vi "ADCP_write_packet_to_serial_port.vi"(8 "error in (no error)":errorcluster, 10 "Packet Bytes":u8[](array[numeric]), 11 "ADCP In":refnum<class "ADCP.lvclass">) -> (0 "error out":errorcluster, 3 "ADCP Out":refnum<class "ADCP.lvclass">)   [LabVIEW 2017, in "ADCP.lvclass"]
uses:
  ADCP.lvclass
  ADCP.lvclass/ADCP.ctl
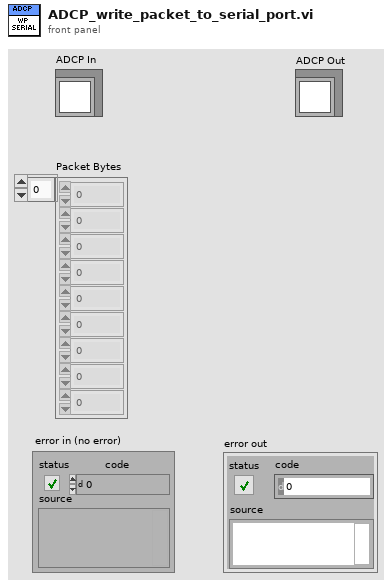
[diagram p1: front panel]
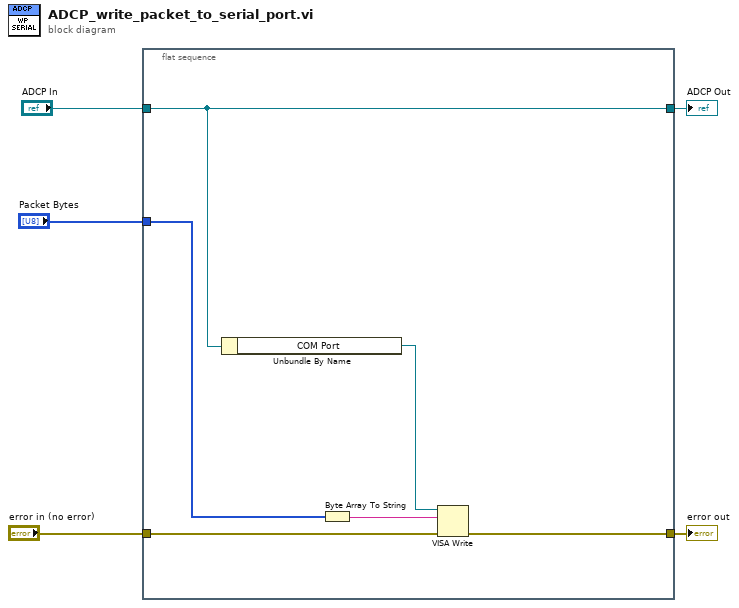
[diagram p0: block diagram]
diagram:
  n1 = flat-sequence {
    tunnel: "error in (no error)" -> [w11]
    tunnel: "ADCP In" -> [w6]
    tunnel: "Packet Bytes" -> [w9]
    tunnel: [w7] -> w1
    tunnel: [w6] -> w2
    frame #0 {
      n2 = Unbundle By Name(w6) -> ("COM Port"=w10:refnum<visa-resource-name>)
      n3 = Byte Array To String(unsigned byte array=w9) -> (string=w8:string)
      n4 = VISA Write(VISA resource name=w10, write buffer=w8, error in (no error)=w11) -> (error out=w7:errorcluster)  [unwired: 2 out]
    }
  }
  "ADCP Out" <- w2
  "error out" <- w1
